vi "Image Processing with Vision Assistant (FPGA)testCount.vi"() -> ()   [LabVIEW 2016]
uses:
  <vilib>/visionFPGA/Controls/IMAQ FPGA Image Size.ctl
  <vilib>/rvi/Emulation/niFpgaSctlEmulationGetInTimedLoop.vi
  <vilib>/rvi/Emulation/niFpgaProcessEmulError.vi
  <vilib>/rvi/Emulation/niFpgaGetClockAttributes.vi
  <vilib>/rvi/Emulation/niFpgaEmulationReportErrorSimple.vi
  <vilib>/rvi/eio/common/nirviEmuTemplateMethod_errors.vi
  <vilib>/rvi/interface/RandomDataEmulation/niFpgaRandomDataHandleErrors.vi
  <vilib>/rvi/DataTransferAndStorage/Container/Common/niFpgaContainerGetUniqueNameForEmu.vi
  <vilib>/rvi/DataTransferAndStorage/Container/Common/niFpgaContainerSetEmuInfo.vi
  <vilib>/rvi/eio/common/nirviEmuReportErrorAndStop.vi
  <vilib>/rvi/DataTransferAndStorage/Container/Common/niFpgaContainerExecOnDevCompGetState.vi
  <vilib>/rvi/Emulation/niFpgaEmulationIsFPGAContextNoSignature.vi
  <vilib>/rvi/errors/niFpgaSetErrorForExecOnDevCompSimple.vi
  <vilib>/rvi/FIFO/Fifo_Resource/nirvififoEmulationSetSize.vi
  <vilib>/rvi/FIFO/Fifo_Resource/nirviFifoEmulationQueueMgr.vi
  <instcachedir>/0/nirviFifoEmulationQueueMgr_E5CAEC123FF24DC58D834DCA3CDAA9B5.lvgen/nirviFifoEmulationQueueMgr_E5CAEC123FF24DC58D834DCA3CDAA9B5_002.vi
  <vilib>/rvi/FIFO/Fifo_Resource/nirvififoEmulationDetermineInputValidOut.vi
  <vilib>/rvi/FIFO/Fifo_Resource/nirvififoEmulationCreateLock.vi
  <vilib>/rvi/FIFO/Fifo_Resource/nirvififoEmulationObtainLock.vi
  <vilib>/rvi/FIFO/Fifo_Resource/nirvififoEmulationReleaseLock.vi
  <vilib>/rvi/occurrence/nirviWaitOnOccurrenceBase.vi
  <vilib>/rvi/errors/nirviReportUnexpectedCaseInternalError.vi
  <vilib>/rvi/errors/nirviReportUnexpectedCaseInternalError (U32).vi
  <vilib>/Utility/error.llb/Clear Errors.vi
  <vilib>/rvi/Emulation/niFpgaCriticalErrorInLSC.vi
  <vilib>/eio/EIONode/EIONode.xnode
  <vilib>/rvi/DataTransferAndStorage/Container/XNode/niFpgaContainer.xnode
  <vilib>/rvi/interface/RandomDataEmulation/nirviRandomDataFpgaReadWriteTemplate.vi
  <vilib>/rvi/LocalResourceManager/LocalResourceManager.xnode
  <vilib>/rvi/FIFO/Fifo_Resource/niFpgaFifoEmulationRefIn.vi
panel:
  out "Numeric":i16
  out "Count":u32
  out "OutputType":u8
  out "CanSendImage":bool=TRUE
  out "Mode LED Status":bool=TRUE
  out "Radio LED Status":bool=TRUE
  out "outputExtreme2":bool=TRUE
  out "outputExtreme1":bool=TRUE
  out "outputDOG2":bool=TRUE
  out "outputDOG1":bool=TRUE
  out "Ready For Output":bool=TRUE
  out "StartOfImage":bool=TRUE
  in  "Image Size":T1={"Width"=640, "Height"=480}
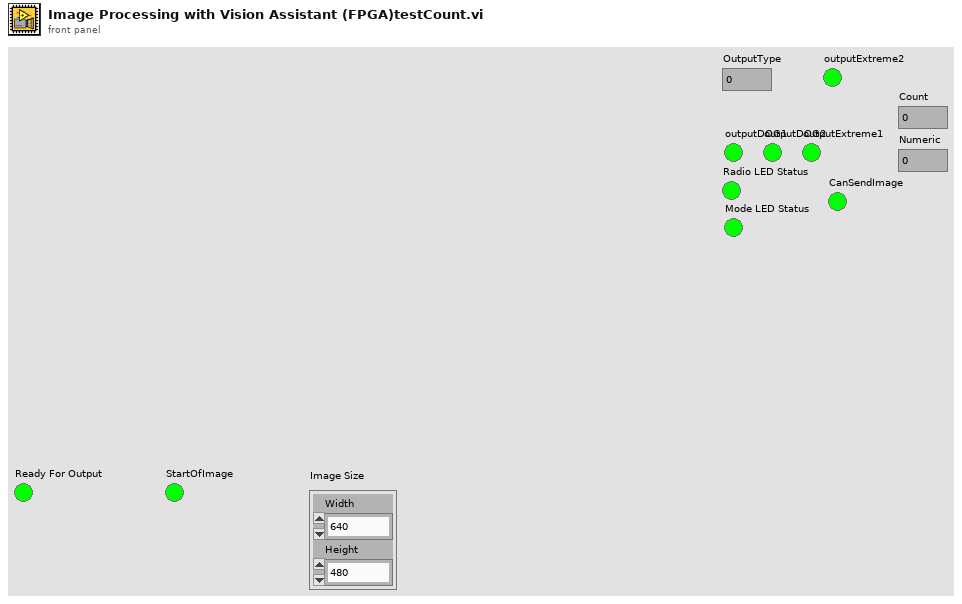
[diagram p1: front panel]
types:
  T1 = typedef "IMAQ FPGA Image Size.ctl" = cluster{"Width":u32, "Height":u32}
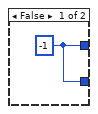
[diagram p10: hidden frame]
diagram:
  # "1. IMAQ FPGA FIFO to Pixel Bus.vi\n    - This VI reads image pixels out of the \"Source Image FIFO\"  Host to Target DMA FIFO that were written by the \"IMAQ FPGA Image Transfer to Target.vi\" function on the host VI.  The pixels are converted into the Pixel Bus format that the Vision Assistant Express VI and the rest of the Vision Development Module FPGA functions use to convey pixel data and image timing information.\n    - Creating a control for the Image Size input allows the \"IMAQ FPGA Configure Image Transfer to Target.vi\" function on the host VI to automatically set the width and height of the image that will be transferred via the FIFO.\n\n2. Vision Assistant Express VI\n    - Use this Express VI to perform the desired processing steps on the image.\n    - To open the Vision Assistant configuration environment, double-click the Vision Assistant Express VI.\n    - By default the Vision Assistant Express VI is configured to add 0 to each pixel, making this example effectively just a pass-through that does not change the source image data.\n    - After opening the Vision Assistant configuration environment, delete the step called \"Delete This Step\" prior to creating your own sequence of processing steps.\n\n3. IMAQ FPGA Pixel Bus to FIFO.vi\n    - This VI writes the image pixel data contained in the Pixel Bus to the \"Dest Image FIFO\" Target to Host DMA FIFO.  These pixels can then be read out of the FIFO using the \"IMAQ FPGA Image Transfer from Target.vi\" function on the host VI."
  n1 = flat-sequence {
    frame #0 {
      w1 = FALSE
      w2 = i16 0
      w3 = TRUE ("Ready For Output")
      "StartOfImage" <- w3
      "Ready For Output" <- w3
      "outputDOG1" <- w1
      "outputDOG2" <- w1
      "outputExtreme1" <- w1
      "outputExtreme2" <- w1
      "Radio LED Status" <- w3
      "Mode LED Status" <- w3
      "CanSendImage" <- w1
      "OutputType" <- w2
      "Count" <- w2
      "Numeric" <- w2
    }
    frame #1 {
      n2 = while "Timed Loop" {
        shift-right: [w10] -> _
        shift-left: _ -> [w14]
        shift-right: [w11] -> _
        shift-left: _ -> [w16]
        stop <- FALSE stop-if-true
        n3 = flat-sequence {
          tunnel: [w85] -> w21
          tunnel: [w84] -> w20
          tunnel: [w78] -> w19
          tunnel: [w77] -> w18
          tunnel: [w76] -> w17
          tunnel: w16 -> [w76]
          tunnel: [w75] -> w15
          tunnel: w14 -> [w75]
          tunnel: [w112] -> w26
          tunnel: [w110] -> w25
          tunnel: [w109] -> w24
          tunnel: [w111] -> w23
          tunnel: w21 -> [w110]
          tunnel: w20 -> [w109]
          tunnel: w19 -> [w112]
          tunnel: w18 -> [w111]
          tunnel: w17 -> [w107]
          tunnel: w15 -> [w106]
          tunnel: [w105] -> w13
          tunnel: [w104] -> w12
          tunnel: [w127] -> w4
          tunnel: [w133] -> w8
          tunnel: [w128] -> w6
          tunnel: [w132] -> w7
          tunnel: [w125] -> w9
          tunnel: w26 -> [w133]
          tunnel: w25 -> [w128]
          tunnel: w24 -> [w132]
          tunnel: w23 -> [w125]
          tunnel: w13 -> [w130]
          tunnel: w12 -> [w131]
          tunnel: [w126] -> w5
          tunnel: w9 -> [w135]
          tunnel: w8 -> [w144]
          tunnel: w7 -> [w140]
          tunnel: w6 -> [w141]
          tunnel: w5 -> [w137]
          tunnel: w4 -> [w136]
          tunnel: [w137] -> w74
          tunnel: [w136] -> w73
          tunnel: [w141] -> w72
          tunnel: [w140] -> w71
          tunnel: [w143] -> w70
          tunnel: [w134] -> w69
          tunnel: [w138] -> w66
          tunnel: w74 -> [w150]
          tunnel: w73 -> [w155]
          tunnel: w72 -> [w152]
          tunnel: w71 -> [w157]
          tunnel: w70 -> [w159]
          tunnel: w69 -> [w158]
          tunnel: [w149] -> w68
          tunnel: [w154] -> w67
          tunnel: w66 -> [w160]
          tunnel: [w150] -> w65
          tunnel: [w155] -> w64
          tunnel: [w152] -> w63
          tunnel: [w157] -> w62
          tunnel: [w156] -> w54
          tunnel: w68 -> [w206]
          tunnel: w67 -> [w205]
          tunnel: w65 -> [w180]
          tunnel: w64 -> [w179]
          tunnel: w63 -> [w181]
          tunnel: w62 -> [w198]
          tunnel: [w184] -> w61
          tunnel: [w178] -> w60
          tunnel: [w180] -> w59
          tunnel: [w179] -> w58
          tunnel: [w181] -> w57
          tunnel: [w198] -> w56
          tunnel: [w203] -> w55
          tunnel: w54 -> [w202]
          tunnel: [w199] -> w53
          tunnel: [w196] -> w52
          tunnel: [w190] -> w51
          tunnel: [w191] -> w50
          tunnel: [w184] -> w49
          tunnel: [w178] -> w48
          tunnel: [w180] -> w11
          tunnel: [w179] -> w10
          tunnel: w61 -> [w247]
          tunnel: w60 -> [w246]
          tunnel: w59 -> [w223]
          tunnel: w58 -> [w245]
          tunnel: w57 -> [w225]
          tunnel: w56 -> [w244]
          tunnel: w55 -> [w241]
          tunnel: w53 -> [w232]
          tunnel: w52 -> [w233]
          tunnel: w51 -> [w231]
          tunnel: w50 -> [w230]
          tunnel: w49 -> [w235]
          tunnel: w48 -> [w236]
          tunnel: [w238] -> w47
          tunnel: [w227] -> w46
          tunnel: [w228] -> w45
          tunnel: [w233] -> w44
          tunnel: [w232] -> w43
          tunnel: [w231] -> w42
          tunnel: [w230] -> w41
          tunnel: w47 -> [w289]
          tunnel: w46 -> [w288]
          tunnel: w45 -> [w287]
          tunnel: w44 -> [w285]
          tunnel: w43 -> [w279]
          tunnel: w42 -> [w284]
          tunnel: w41 -> [w281]
          tunnel: [w286] -> w40
          tunnel: [w281] -> w39
          tunnel: [w284] -> w38
          tunnel: [w279] -> w37
          tunnel: [w285] -> w36
          tunnel: [w282] -> w35
          tunnel: [w278] -> w34
          tunnel: w40 -> [w315]
          tunnel: w39 -> [w305]
          tunnel: w38 -> [w311]
          tunnel: w37 -> [w307]
          tunnel: w36 -> [w310]
          tunnel: w35 -> [w314]
          tunnel: w34 -> [w313]
          tunnel: [w309] -> w33
          tunnel: [w304] -> w32
          tunnel: [w312] -> w31
          tunnel: [w305] -> w30
          tunnel: [w311] -> w29
          tunnel: [w307] -> w28
          tunnel: [w310] -> w27
          tunnel: w33 -> [w340]
          tunnel: w32 -> [w339]
          tunnel: w31 -> [w338]
          tunnel: w30 -> [w332]
          tunnel: w29 -> [w331]
          tunnel: w28 -> [w334]
          tunnel: w27 -> [w337]
          tunnel: [w332] -> _
          tunnel: [w331] -> _
          frame #0 {
            n4 = xnode ("FIFO Get Number of Elements to Read")() -> ("Number of Elements to Read"=w80:u32)  [unwired: 1 in, 1 out]
            n5 = Unbundle By Name("Image Size") -> ("Width"=w85:u32, "Height"=w84:u32)
            n6 = local read "Mode LED Status"() -> (w83:bool)
            n7 = local read "Radio LED Status"() -> (w81:bool)
            n8 = Greater Than 0?(x=w80) -> (x > 0?=w79:bool)
            n9 = case shown="True" w79 {
              selector: w79 -> [w87 w89]
              tunnel: [_ w90] -> w78
              tunnel: [w87 w89] -> w77
              frame False {
              }
              frame True {
                n10 = flat-sequence {
                  tunnel: [w98] -> w88
                  tunnel: w88 -> [w100]
                  frame #0 {
                    n11 = local read "Numeric"() -> (w99:i16)
                    n12 = Increment(x=w99) -> (x+1=w98:i16)
                    n13 = local write "Numeric"(w98) -> ()
                  }
                  frame #1 {
                    n14 = xnode ("FIFO Write")("Element"=w100, "Timeout"=0) -> ()  [unwired: 1 in, 2 out]
                  }
                  frame #2 {
                    n15 = call "Tick Count"() -> ("Tick Count(uSec)"=w103:u32)
                    n16 = xnode ("FIFO Write")("Element"=w103, "Timeout"=0) -> ()  [unwired: 1 in, 2 out]
                  }
                }
                n17 = xnode ("FIFO Read")("Timeout"=0) -> ("Element"=w97:u32)  [unwired: 1 in, 2 out]
                n18 = Split Number(x=w97) -> (hi(x)=w95:u16, lo(x)=w96:u16)
                n19 = Split Number(x=w95) -> (lo(x)=w94:u8)  [unwired: 1 out]
                n20 = Split Number(x=w96) -> (hi(x)=w93:u8, lo(x)=w92:u8)
                n21 = call "To Gray_FPGA (SubVI)-RGB.vi"("B"=w92, "G"=w93, "R"=w94) -> ("Data Out"=w90:fxp<+,8,8>)  [unwired: 8 in]
              }
            }
            n22 = Not(x=w83) -> (.not. x?=w82:bool)
            n23 = xnode "FPGA I/O Node"("Radio LED Green"=w81) -> ()  [unwired: 1 in, 1 out]
            n24 = xnode "FPGA I/O Node"("Mode LED Green"=w83) -> ()  [unwired: 1 in, 1 out]
            n25 = xnode "FPGA I/O Node"("Mode LED Red"=w82) -> ()  [unwired: 1 in, 1 out]
          }
          frame #1 {
            n26 = Decrement(x=w109) -> (x-1=w115:u32)
            n27 = Decrement(x=w110) -> (x-1=w114:u32)
            n28 = local read "StartOfImage"() -> (w108:bool)
            n29 = Equal?(x=w106, y=w115) -> (x = y?=w117:bool)
            n30 = Equal?(x=w107, y=w114) -> (x = y?=w116:bool)
            n31 = And(x=w117, y=w116) -> (x .and. y?=w113:bool)
            n32 = case shown="True" w113 {
              frame False {
              }
              frame True {
                # "当接收完最后一个像素时，由于后续差分未做完，\n停止接收，Ready For Output置为F"
                n33 = local write "Ready For Output"(FALSE ("Ready For Output")) -> ()
              }
            }
            n34 = case shown="True" w108 {
              selector: w108 -> [_ w121]
              tunnel: w107 -> [w119 _]
              tunnel: w106 -> [w118 _]
              tunnel: [w119 i16 -1] -> w105
              tunnel: [w118 w120] -> w104
              frame False {
              }
              frame True {
                w120 = i16 0
                n35 = Not(x=w121) -> (.not. x?=w122:bool)
                n36 = local write "Numeric"(w120) -> ()
                n37 = local write "StartOfImage"(w122) -> ()
                n38 = local write "Ready For Output"(w121) -> ()
                n39 = local write "CanSendImage"(w121) -> ()
                n40 = local write "Count"(w120) -> ()
              }
            }
          }
          frame #2 {
            n41 = local read "Ready For Output"() -> (w129:bool)
            n42 = call "Cal ColNum(SubVI) - rgb.vi"("Ready For Input"=w129, "DV"=w125, "Width"=w128, "preCol"=w130) -> ("curCol"=w126:u16)  [unwired: 7 in]
            n43 = call "Cal RowNum(SubVI) - rgb.vi"("Width"=w128, "preRow"=w131, "preCol"=w130) -> ("curRow"=w127:u16)  [unwired: 8 in]
          }
          frame #3 {
            # "第一组第一层高斯滤波"
            n44 = xnode "1-1 Gaussianed cached Memory"() -> ("Memory Out"=w138:refnum<k21>)
            n45 = xnode "1-1 pixel cached Memory"() -> ("Memory Out"=w142:refnum<k21>)
            n46 = call "DOG.vi"("Gaussianed cached Memory"=w138, "pixel cached Memory"=w142, "preGaussianed cached Memory"=w138, "Data in"=w144, "DV in"=w135, "Height"=w140, "Width"=w141, "DelayRowCount"=i16 0, "Rows"=w136, "Cols"=w137) -> ("GaussianFilterData out"=w143:fxp<+,12,12>, "DV out"=w134:bool)  [unwired: 6 in, 2 out]
            n47 = case shown="True" w134 {
              tunnel: w143 -> [_ w146]
              frame False {
              }
              frame True {
                n48 = local read "OutputType"() -> (w145:u8)
                n49 = case shown="1" w145 {
                  tunnel: w146 -> [_ w147]
                  frame 0, Default {
                  }
                  frame 1 {
                    # "第一组第一层滤波图像"
                    n50 = xnode ("FIFO Write")("Element"=w147, "Timeout"=0) -> ()  [unwired: 1 in, 2 out]
                  }
                }
              }
            }
          }
          frame #4 {
            # "第一组第二层高斯滤波"
            n51 = xnode "1-2 Gaussianed cached Memory"() -> ("Memory Out"=w156:refnum<k21>)
            n52 = xnode "1-2 pixel cached Memory"() -> ("Memory Out"=w161:refnum<k21>)
            n53 = call "DOG.vi"("Gaussianed cached Memory"=w156, "pixel cached Memory"=w161, "preGaussianed cached Memory"=w160, "Data in"=w159, "DV in"=w158, "Height"=w157, "Width"=w152, "DelayRowCount"=i16 2, "Rows"=w155, "Cols"=w150) -> ("out Row"=w151:u16, "GaussianFilterData out"=w154:fxp<+,12,12>, "DV out"=w149:bool, "DOG Out"=w153:fxp<+/-,13,13>)  [unwired: 6 in]
            n54 = case shown="True" w149 {
              selector: w149 -> [_ w166]
              tunnel: w154 -> [_ w173]
              tunnel: w153 -> [_ w164]
              tunnel: w152 -> [_ w172]
              tunnel: w151 -> [_ w171]
              tunnel: w150 -> [_ w170]
              frame False {
              }
              frame True {
                # "第一组第一层和第二层差分"
                n55 = call "calcAddressInMemory.vi"("Width"=w172, "Rows"=w171, "Cols"=w170, "divider"=u8 8) -> ("addressInMemory"=w168:u16)  [unwired: 5 in]
                n56 = local read "OutputType"() -> (w165:u8)
                n57 = local read "outputDOG1"() -> (w163:bool)
                n58 = call "putFilterPixeltoMemory(I8).vi"("DV in"=w166, "addressInMemory"=w168, "Data In"=w164, "Memory in"=refnum<k21> "DOG1-1") -> ()  [unwired: 8 in]
                n59 = case shown="2" w165 {
                  tunnel: w173 -> [_ w176]
                  frame 0, Default {
                  }
                  frame 2 {
                    # "第一组第二层滤波图像"
                    n60 = xnode ("FIFO Write")("Element"=w176, "Timeout"=0) -> ()  [unwired: 1 in, 2 out]
                  }
                }
                n61 = case shown="True" w163 {
                  tunnel: w164 -> [_ w175]
                  frame False {
                  }
                  frame True {
                    n62 = xnode ("FIFO Write")("Element"=w175, "Timeout"=0) -> ()  [unwired: 1 in, 2 out]
                  }
                }
              }
            }
          }
          frame #5 {
            w197 = u32 2 ("y")
            # "第一组第三层高斯滤波"
            n63 = xnode "1-3 pixel cached Memory"() -> ("Memory Out"=w204:refnum<k21>)
            n64 = xnode "1-3 Gaussianed cached Memory"() -> ("Memory Out"=w203:refnum<k21>)
            n65 = Subtract(x=w179, y=i16 6) -> (x-y=w187:u16)
            n66 = Quotient & Remainder(x=w180, y=w197) -> (x-y*floor(x/y)=w186:u32, floor(x/y)=w188:u32)
            n67 = Quotient & Remainder(x=w187, y=w197) -> (x-y*floor(x/y)=w185:u32, floor(x/y)=w189:u32)
            n68 = Quotient & Remainder(x=w181, y=w197) -> (floor(x/y)=w199:u32)  [unwired: 1 out]
            n69 = Quotient & Remainder(x=w198, y=w197) -> (floor(x/y)=w196:u32)  [unwired: 1 out]
            n70 = call "DOG.vi"("Gaussianed cached Memory"=w203, "pixel cached Memory"=w204, "preGaussianed cached Memory"=w202, "Data in"=w205, "DV in"=w206, "Height"=w198, "Width"=w181, "DelayRowCount"=i16 4, "Rows"=w179, "Cols"=w180) -> ("out Row"=w182:u16, "GaussianFilterData out"=w184:fxp<+,12,12>, "DV out"=w178:bool, "DOG Out"=w183:fxp<+/-,13,13>)  [unwired: 6 in]
            n71 = Equal To 0?(x=w186) -> (x = 0?=w195:bool)
            n72 = Equal To 0?(x=w185) -> (x = 0?=w194:bool)
            n73 = Greater Or Equal To 0?(x=w187) -> (x >= 0?=w193:bool)
            n74 = Compound Arithmetic op=AND(w195, w194, w193) -> (w192:bool)
            n75 = case shown="True" w178 {
              selector: w178 -> [_ w211]
              tunnel: w184 -> [_ w219]
              tunnel: w183 -> [_ w212]
              tunnel: w182 -> [_ w215]
              tunnel: w181 -> [_ w214]
              tunnel: w180 -> [_ w213]
              frame False {
              }
              frame True {
                # "第一组第二层和第三层差分"
                n76 = call "calcAddressInMemory.vi"("Width"=w214, "Rows"=w215, "Cols"=w213, "divider"=u8 6) -> ("addressInMemory"=w217:u16)  [unwired: 5 in]
                n77 = local read "OutputType"() -> (w210:u8)
                n78 = call "putFilterPixeltoMemory(I8).vi"("DV in"=w211, "addressInMemory"=w217, "Data In"=w212, "Memory in"=refnum<k21> "DOG1-2") -> ()  [unwired: 8 in]
                n79 = case shown="3" w210 {
                  tunnel: w219 -> [_ w220]
                  frame 0, Default {
                  }
                  frame 3 {
                    # "第一组第三层滤波图像"
                    n80 = xnode ("FIFO Write")("Element"=w220, "Timeout"=0) -> ()  [unwired: 1 in, 2 out]
                  }
                }
              }
            }
            n81 = case shown="True" w192 {
              tunnel: [w207 w209] -> w191
              tunnel: w188 -> [_ w209]
              tunnel: [w207 w208] -> w190
              tunnel: w189 -> [_ w208]
              frame False {
                w207 = i16 -1 ("t")
              }
              frame True {
              }
            }
          }
          frame #6 {
            w229 = i16 0 ("delayRowCount")
            # "第二组第一层高斯滤波"
            # "第一组第四层高斯滤波"
            n82 = xnode "2-1 Gaussianed cached Memory"() -> ("Memory Out"=w238:refnum<k21>)
            n83 = xnode "2-1 pixel cached Memory"() -> ("Memory Out"=w234:refnum<k21>)
            n84 = xnode "1-4 pixel cached Memory"() -> ("Memory Out"=w242:refnum<k21>)
            n85 = xnode "1-4 Gaussianed cached Memory"() -> ("Memory Out"=w243:refnum<k21>)
            n86 = call "Gaussian Filter(Pic1 LevelOther).vi"("Height"=w233, "Width"=w232, "Rows"=w231, "Cols"=w230, "Memory in"=w234, "Data in"=w235, "DV in"=w236, "DelayRowCount"=w229) -> ("DV out"=w228:bool, "Data Out"=w227:fxp<+,8,8>)  [unwired: 5 in, 1 out]
            n87 = call "DOG.vi"("Gaussianed cached Memory"=w243, "pixel cached Memory"=w242, "preGaussianed cached Memory"=w241, "Data in"=w247, "DV in"=w246, "Height"=w244, "Width"=w225, "DelayRowCount"=i16 6, "Rows"=w245, "Cols"=w223) -> ("out Row"=w224:u16, "GaussianFilterData out"=w237:fxp<+,12,12>, "DV out"=w222:bool, "DOG Out"=w226:fxp<+/-,13,13>)  [unwired: 6 in]
            n88 = call "calcAddressInMemory.vi"("Width"=w232, "Rows"=w231, "delayRowCount"=w229, "Cols"=w230) -> ("addressInMemory"=w239:u16)  [unwired: 5 in]
            n89 = call "putFilterPixeltoMemory.vi"("Data In"=w227, "DV in"=w228, "addressInMemory"=w239, "Memory in"=w238) -> ()
            n90 = case shown="True" w228 {
              tunnel: w227 -> [_ w249]
              frame False {
              }
              frame True {
                # "第二组第一层滤波图像"
                n91 = local read "OutputType"() -> (w248:u8)
                n92 = case shown="5" w248 {
                  tunnel: w249 -> [_ w250]
                  frame 0, Default {
                  }
                  frame 5 {
                    n93 = xnode ("FIFO Write")("Element"=w250, "Timeout"=0) -> ()  [unwired: 1 in, 2 out]
                  }
                }
              }
            }
            n94 = case shown="True" w222 {
              selector: w222 -> [_ w262]
              tunnel: w237 -> [_ w266]
              tunnel: w226 -> [_ w263]
              tunnel: w225 -> [_ w261]
              tunnel: w224 -> [_ w255]
              tunnel: w223 -> [_ w256]
              frame False {
              }
              frame True {
                w258 = refnum<k21> "DOG1-3" ("Memory in")
                # "第一组第三层和第四层差分"
                n95 = local read "outputExtreme1"() -> (w253:bool)
                n96 = local read "OutputType"() -> (w257:u8)
                n97 = call "calcAddressInMemory.vi"("Width"=w261, "Rows"=w255, "Cols"=w256, "divider"=u8 4) -> ("addressInMemory"=w264:u16)  [unwired: 5 in]
                n98 = case shown="4" w257 {
                  tunnel: w266 -> [_ w277]
                  frame 0, Default {
                  }
                  frame 4 {
                    # "第一组第四层滤波图像"
                    n99 = xnode ("FIFO Write")("Element"=w277, "Timeout"=0) -> ()  [unwired: 1 in, 2 out]
                  }
                }
                n100 = call "putFilterPixeltoMemory(I8).vi"("DV in"=w262, "addressInMemory"=w264, "Data In"=w263, "Memory in"=w258) -> ()  [unwired: 8 in]
                n101 = call "detectAndTransExtremePoint.vi"("Col"=w256, "Row"=w255, "Level3 Memory"=w258, "Level2 Memory"=refnum<k21> "DOG1-2" ("Memory In"), "Level1 Memory"=refnum<k21> "DOG1-1" ("Memory In"), "Width"=w261) -> ("isExtreme?"=w252:bool)  [unwired: 5 in]
                n102 = And(x=w252, y=w253) -> (x .and. y?=w254:bool)
                n103 = case shown="True" w254 {
                  tunnel: w255 -> [_ w274]
                  tunnel: w256 -> [_ w268]
                  frame False {
                  }
                  frame True {
                    w267 = refnum<k21> "extreme FIFO"  # FIFO
                    n104 = Subtract(x=w274, y=u16 2) -> (x-y=w272:u16)
                    n105 = xnode ("FIFO Write")("Element"=w272, "Timeout"=0, "FIFO In"=w267) -> ("FIFO Out"=w270:refnum<k21>)  [unwired: 1 out]
                    n106 = Increment(x=w268) -> (x+1=w269:u16)
                    n107 = xnode ("FIFO Write")("Element"=w269, "Timeout"=0, "FIFO In"=w270) -> ()  [unwired: 2 out]
                  }
                }
              }
            }
          }
          frame #7 {
            # "第二组第二层高斯滤波"
            n108 = xnode "2-2 Gaussianed cached Memory"() -> ("Memory Out"=w286:refnum<k21>)
            n109 = xnode "2-2 pixel cached Memory"() -> ("Memory Out"=w290:refnum<k21>)
            n110 = call "DOG.vi"("Gaussianed cached Memory"=w286, "pixel cached Memory"=w290, "preGaussianed cached Memory"=w289, "Data in"=w288, "DV in"=w287, "Height"=w285, "Width"=w279, "DelayRowCount"=i16 2, "Rows"=w284, "Cols"=w281) -> ("out Row"=w280:u16, "GaussianFilterData out"=w282:fxp<+,12,12>, "DV out"=w278:bool, "DOG Out"=w283:fxp<+/-,13,13>)  [unwired: 6 in]
            n111 = case shown="True" w278 {
              selector: w278 -> [_ w293]
              tunnel: w283 -> [_ w294]
              tunnel: w282 -> [_ w301]
              tunnel: w281 -> [_ w297]
              tunnel: w280 -> [_ w296]
              tunnel: w279 -> [_ w295]
              frame False {
              }
              frame True {
                # "第二组第一层和第二层差分"
                n112 = call "calcAddressInMemory.vi"("Width"=w295, "Rows"=w296, "Cols"=w297, "divider"=u8 8) -> ("addressInMemory"=w299:u16)  [unwired: 5 in]
                n113 = local read "OutputType"() -> (w292:u8)
                n114 = call "putFilterPixeltoMemory(I8).vi"("DV in"=w293, "addressInMemory"=w299, "Data In"=w294, "Memory in"=refnum<k21> "DOG2-1") -> ()  [unwired: 8 in]
                n115 = case shown="6" w292 {
                  tunnel: w301 -> [_ w302]
                  frame 0, Default {
                  }
                  frame 6 {
                    # "第二组第二层滤波图像"
                    n116 = xnode ("FIFO Write")("Element"=w302, "Timeout"=0) -> ()  [unwired: 1 in, 2 out]
                  }
                }
              }
            }
          }
          frame #8 {
            # "第二组第三层高斯滤波"
            n117 = xnode "2-3 Gaussianed cached Memory"() -> ("Memory Out"=w312:refnum<k21>)
            n118 = xnode "2-3 pixel cached Memory"() -> ("Memory Out"=w316:refnum<k21>)
            n119 = call "DOG.vi"("Gaussianed cached Memory"=w312, "pixel cached Memory"=w316, "preGaussianed cached Memory"=w315, "Data in"=w314, "DV in"=w313, "Height"=w310, "Width"=w307, "DelayRowCount"=i16 4, "Rows"=w311, "Cols"=w305) -> ("out Row"=w306:u16, "GaussianFilterData out"=w309:fxp<+,12,12>, "DV out"=w304:bool, "DOG Out"=w308:fxp<+/-,13,13>)  [unwired: 6 in]
            n120 = case shown="True" w304 {
              selector: w304 -> [_ w319]
              tunnel: w309 -> [_ w327]
              tunnel: w308 -> [_ w320]
              tunnel: w307 -> [_ w323]
              tunnel: w306 -> [_ w322]
              tunnel: w305 -> [_ w321]
              frame False {
              }
              frame True {
                # "第二组第二层和第三层差分"
                n121 = local read "OutputType"() -> (w318:u8)
                n122 = call "calcAddressInMemory.vi"("Width"=w323, "Rows"=w322, "Cols"=w321, "divider"=u8 6) -> ("addressInMemory"=w325:u16)  [unwired: 5 in]
                n123 = case shown="7" w318 {
                  tunnel: w327 -> [_ w329]
                  frame 0, Default {
                  }
                  frame 7 {
                    # "第二组第三层滤波图像"
                    n124 = xnode ("FIFO Write")("Element"=w329, "Timeout"=0) -> ()  [unwired: 1 in, 2 out]
                  }
                }
                n125 = call "putFilterPixeltoMemory(I8).vi"("DV in"=w319, "addressInMemory"=w325, "Data In"=w320, "Memory in"=refnum<k21> "DOG2-2") -> ()  [unwired: 8 in]
              }
            }
          }
          frame #9 {
            # "第二组第四层高斯滤波"
            n126 = xnode "2-4 Gaussianed cached Memory"() -> ("Memory Out"=w341:refnum<k21>)
            n127 = xnode "2-4 pixel cached Memory"() -> ("Memory Out"=w342:refnum<k21>)
            n128 = call "DOG.vi"("Gaussianed cached Memory"=w341, "pixel cached Memory"=w342, "preGaussianed cached Memory"=w338, "Data in"=w340, "DV in"=w339, "Height"=w337, "Width"=w334, "DelayRowCount"=i16 6, "Rows"=w331, "Cols"=w332) -> ("out Row"=w333:u16, "GaussianFilterData out"=w336:fxp<+,12,12>, "DV out"=w330:bool, "DOG Out"=w335:fxp<+/-,13,13>)  [unwired: 6 in]
            n129 = case shown="True" w330 {
              selector: w330 -> [_ w356]
              tunnel: w336 -> [_ w362]
              tunnel: w335 -> [_ w355]
              tunnel: w334 -> [_ w354]
              tunnel: w333 -> [_ w352]
              tunnel: w332 -> [_ w353]
              frame False {
              }
              frame True {
                w357 = refnum<k21> "DOG2-3" ("Memory in")
                # "第二组第三层和第四层差分"
                n130 = local read "OutputType"() -> (w348:u8)
                n131 = local read "outputExtreme2"() -> (w349:bool)
                n132 = call "calcAddressInMemory.vi"("Width"=w354, "Rows"=w352, "Cols"=w353, "divider"=u8 4) -> ("addressInMemory"=w360:u16)  [unwired: 5 in]
                n133 = case shown="8" w348 {
                  tunnel: w362 -> [_ w364]
                  frame 0, Default {
                  }
                  frame 8 {
                    # "第二组第四层滤波图像"
                    n134 = xnode ("FIFO Write")("Element"=w364, "Timeout"=0) -> ()  [unwired: 1 in, 2 out]
                  }
                }
                n135 = local read "Count"() -> (w347:u32)
                n136 = call "putFilterPixeltoMemory(I8).vi"("DV in"=w356, "addressInMemory"=w360, "Data In"=w355, "Memory in"=w357) -> ()  [unwired: 8 in]
                n137 = Increment(x=w347) -> (x+1=w346:u32)
                n138 = local write "Count"(w346) -> ()
                n139 = call "detectAndTransExtremePoint.vi"("Col"=w353, "Row"=w352, "Level3 Memory"=w357, "Level2 Memory"=refnum<k21> "DOG2-2" ("Memory In"), "Level1 Memory"=refnum<k21> "DOG2-1" ("Memory In"), "Width"=w354) -> ("isExtreme?"=w350:bool)  [unwired: 5 in]
                n140 = Not And(1:w349, 2:w350) -> (0:w351:bool)
                n141 = case shown="True" w351 {
                  tunnel: w352 -> [_ w372]
                  tunnel: w353 -> [_ w366]
                  frame False {
                  }
                  frame True {
                    w365 = refnum<k21> "extreme FIFO dec"  # FIFO
                    n142 = Subtract(x=w372, y=u16 2) -> (x-y=w370:u16)
                    n143 = xnode ("FIFO Write")("Element"=w370, "Timeout"=0, "FIFO In"=w365) -> ("FIFO Out"=w368:refnum<k21>)  [unwired: 1 out]
                    n144 = Increment(x=w366) -> (x+1=w367:u32)
                    n145 = xnode ("FIFO Write")("Element"=w367, "Timeout"=0, "FIFO In"=w368) -> ()  [unwired: 2 out]
                  }
                }
              }
            }
            n146 = case shown="True" w330 {
              frame False {
              }
              frame True {
                n147 = flat-sequence {
                  frame #0 {
                    n148 = call "Tick Count9"() -> ("Tick Count(uSec)"=w345:u32)
                    n149 = xnode ("FIFO Write")("Element"=w345, "Timeout"=0) -> ()  [unwired: 1 in, 2 out]
                  }
                }
              }
            }
          }
        }
      }
    }
  }
